vi "Run Bitfile.vi"() -> ()   [LabVIEW 2011]
uses:
  <vilib>/Platform/TimedLoop/XDataNode/timing_clust.ctl
  <vilib>/Platform/TimedLoop/XDataNode/nitl_modes.ctl
  <vilib>/Platform/TimedLoop/XDataNode/wakeup.ctl
  <vilib>/FPGAPlugInAG/sbRIO-9606/niLvFpga_Open_sbRIO-9606.vi
  <vilib>/rvi/interface/common/dynamic/niFpgaDynamicAddResources.vi
  <vilib>/Utility/error.llb/Error Cluster From Error Code.vi
  <vilib>/rvi/errors/niLvFpgaAdjustHostInterfaceError.vi
  <vilib>/FPGAPlugInAG/Dynamic/niLvFpga_Close_Dynamic.vi
  <vilib>/Platform/TimedLoop/XDataNode/XDataNode.xnode
  <vilib>/rvi/interface/nirviOpenFPGA/nirviOpenFPGA.xnode
  FPGA Bitfiles/natcar_FPGATarget_Top-Level_610FB000.lvbitx
  <vilib>/rvi/interface/nirviReadWriteControl/nirviReadWriteControl.xnode
  <vilib>/rvi/interface/nirviCloseFPGA/nirviCloseFPGA.xnode
  NiFpgaLv.dll
  <vilib>/rvi/interface/Simulation/niFpgaSimulationCallBeginRW.vi
  <vilib>/Platform/TimedLoop/XDataNode/XDNodeRunTimeDep.lvlib
panel:
  out "Vdiff":i32
  out "Vx":dbl
  out "Error":errorcluster
  out "Velocity counts":u32
  out "SC":u16
  out "S5":u16
  out "S4":u16
  out "S3":u16
  out "S2":u16
  out "S1":u16
  out "error":i32
  out "error":i32(graph)
  out "raw L":u16(graph)
  out "raw R":u16(graph)
  in  "manual throttle":bool
  in  "manual steering":bool
  in  "Steering ON 1e-7s":u32=15000
  in  "Steering frequency (Hz)":u16=50
  in  "GO duty (100*%)":u16
  in  "GO frequency (Hz)":u16=200
  out "Steering duty (cycles)":u32
  out "L":u32
  out "R":u32
  in  "uBlaze Reset":bool
  in  "stop":bool
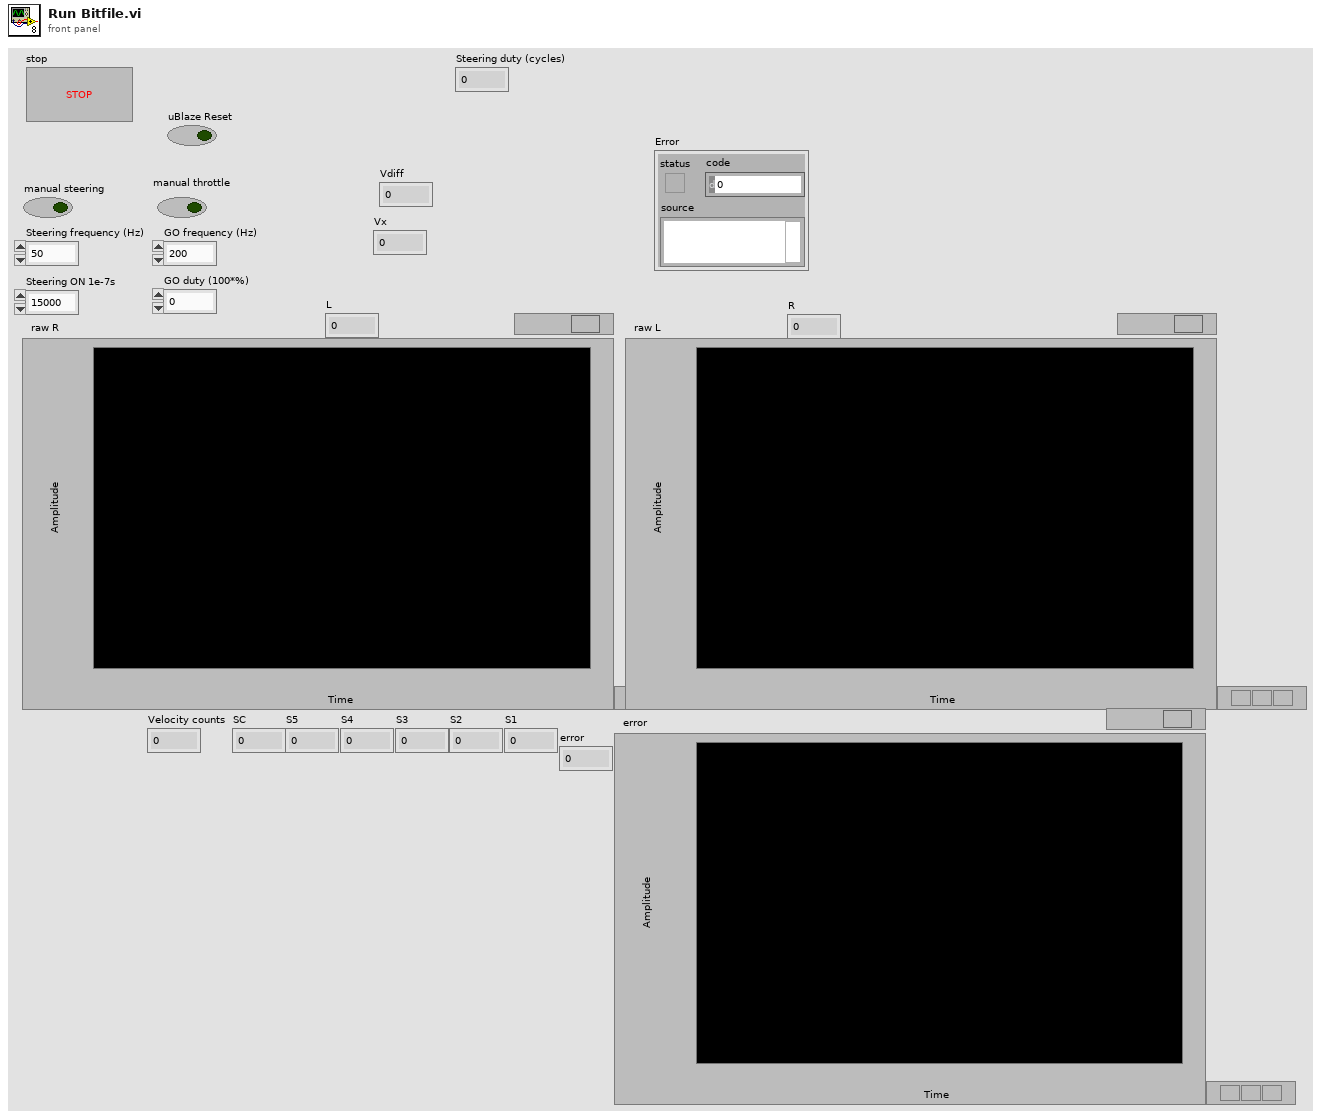
[diagram p1: front panel]
types:
  T1 = typedef "XDNodeRunTimeDep.lvlib/timing_clust.ctl" = cluster{"Expected End [f-1]":u64, "Actual End [f-1]":u64, "Finished Late? [f-1]":bool, "Expected End [i-1]":u64, "Actual End [i-1]":u64, "Finished Late? [i-1]":bool, "Expected Start [i]":u64, "Actual Start [i]":u64, "Expected Start [f]":u64, "Actual Start [f]":u64, "Source Name":string, "Structure Name":string, "Period":i64, "Deadline":i64, "Offset":i64, "Start":i64, "Priority":i32, "Timeout":i32, "Mode":T2, "Wakeup Reason":T3, "Error":errorcluster, "Source Type":string, "Secondary Source Type":string, "Global End Time":u64, "Global Start Time":u64, "Frame Duration":u64, "Iteration Duration":u64, "Assigned CPU":i32, "I/O Scan Engine Mode":u32}
  T2 = typedef "XDNodeRunTimeDep.lvlib/nitl_modes.ctl" = enum32{"No Change", "Process missed periods, maintain original phase", "Discard missed periods, maintain original phase", "Process missed periods, ignore original phase", "Discard missed periods, ignore original phase"}
  T3 = typedef "XDNodeRunTimeDep.lvlib/wakeup.ctl" = enum32{"Normal", "Aborted", "Asynchronous wakeup", "Timing source error", "Timed loop error", "Timeout"}
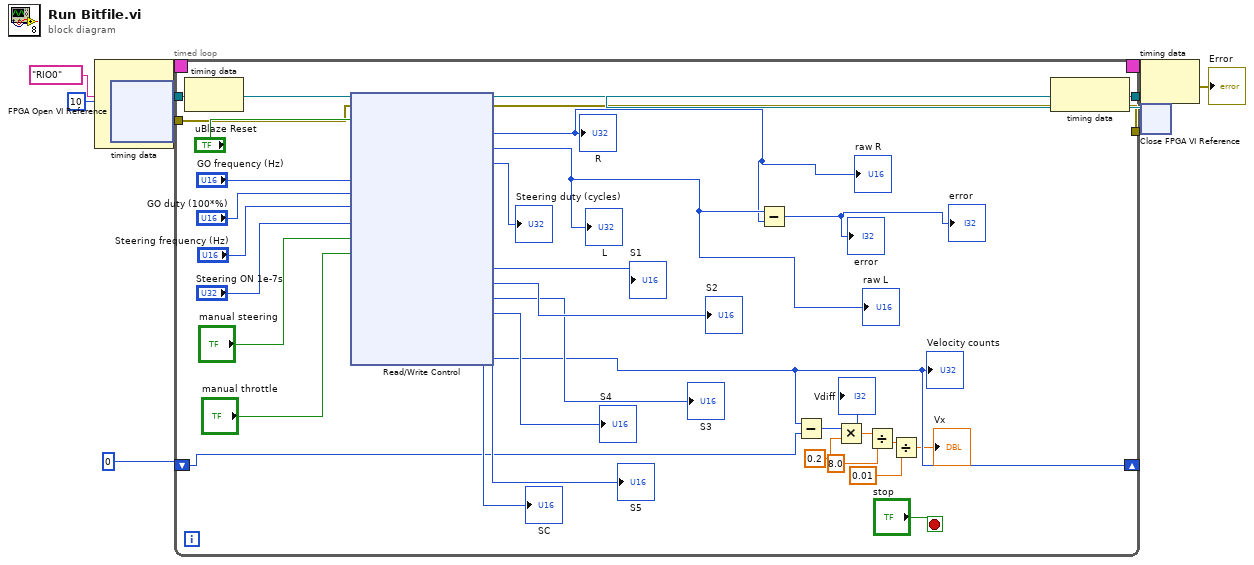
[diagram p0: block diagram]
diagram:
  n1 = node-c288(i64 10 ("Period")) -> (w5:T1)  [unwired: 3 in]
  n2 = xnode "FPGA Open VI Reference"("resource name"=tag "RIO0") -> ("FPGA VI Reference Out"=w10:refnum<k20>, "error out"=w8:errorcluster)  [unwired: 1 in]
  n3 = timed-loop {
    tunnel: w10 -> [w40]
    tunnel: [w39] -> w9
    tunnel: w8 -> [w37]
    tunnel: [w36] -> w7
    timing: w5 -> [_]
    timing-out: [_] -> w4
    shift-right: [w19] -> _
    shift-left: u32 0 ("Velocity counts") -> [w18]
    stop <- "stop" stop-if-true
    n4 = node-c288() -> ()  [unwired: 1 in, 1 out]
    n5 = xnode "Read/Write Control"("FPGA VI Reference In"=w40, "error in"=w37, "uBlaze Reset"="uBlaze Reset", "GO frequency (Hz)"="GO frequency (Hz)", "GO duty (100*%)"="GO duty (100*%)", "Steering frequency (Hz)"="Steering frequency (Hz)", "Steering ON 1e-7s"="Steering ON 1e-7s", "manual steering"="manual steering", "manual throttle"="manual throttle") -> ("FPGA VI Reference Out"=w39:refnum<k20>, "error out"=w36:errorcluster, "AI0"=w27:u16, "AI1"=w28:u16, "Steering duty (cycles)"=→"Steering duty (cycles)":u32, "AI2"=→"S1":u16, "AI3"=→"S2":u16, "AI4"=→"S3":u16, "AI5"=→"S4":u16, "AI6"=→"S5":u16, "AI7"=→"SC":u16, "Velocity counts"=w19:u32)
    "R" <- w27
    "L" <- w28
    "raw R" <- w27
    "raw L" <- w28
    "Velocity counts" <- w19
    n6 = Subtract(x=w28, y=w27) -> (x-y=→"error" →"error":i32)
    n7 = Subtract(x=w19, y=w18) -> (x-y=w17:i32)
    "Vdiff" <- w17
    n8 = Multiply(x=w17, y=0.2) -> (x*y=w15:dbl)
    n9 = Divide(x=w15, y=8.0) -> (x/y=w13:dbl)
    n10 = Divide(x=w13, y=0.01) -> (x/y=→"Vx":dbl)
    n11 = node-c288() -> ()  [unwired: 1 in, 1 out]
  }
  n12 = node-c288(w4) -> (→"Error":errorcluster)
  n13 = xnode "Close FPGA VI Reference"("FPGA VI Reference In"=w9, "error in"=w7) -> ()  [unwired: 1 out]
